vi "Shooter Pneumatics.vi"(10 "Boolean":bool, 11 "Enum":enum16{"Start", "Run", "End"}(ring)=enum."Run") -> (3 "Shooter Angle":T1)   [LabVIEW 2012]
uses:
  <vilib>/Rock Robotics/WPI/Solenoid/WPI_SolenoidChannel.ctl
  <vilib>/Rock Robotics/SystemInterfaces/Typedef/FPGA_TypedefSolenoidModule.ctl
  <vilib>/Rock Robotics/WPI/Solenoid/WPI_SolenoidValue.ctl
  <vilib>/Rock Robotics/WPI/Solenoid/WPI_SolenoidOpenDouble.vi
  <vilib>/Rock Robotics/WPI/Solenoid/WPI_SolenoidSetEnum.vi
panel:
  in  "Solenoid Module 1":T4={"Shoot FWD"=enum."Solenoid 1", "Shoot REV"=enum."Solenoid 2", "Climber"=enum."Solenoid 3", "Climber"=enum."Solenoid 4", "Arm Lock"=enum."Solenoid 5", "Unassigned"=enum."Solenoid 6", "Color"=enum."Solenoid 7", "Unassigned"=enum."Solenoid 8", "Module"=enum."Solenoid Module 1"}
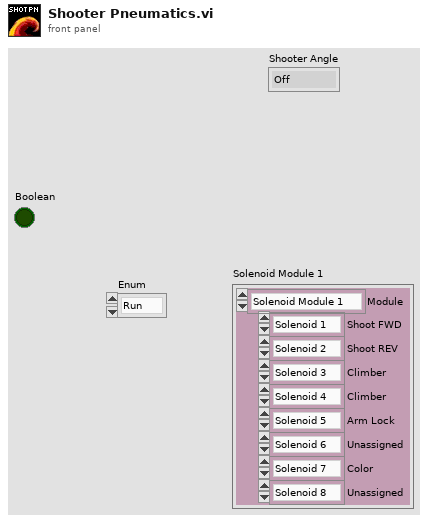
[diagram p1: front panel]
types:
  T1 = typedef "WPI_SolenoidValue.ctl" = enum16{"Off", "On", "Forward", "Reverse"}
  T2 = typedef "WPI_SolenoidChannel.ctl" = enum8{"Solenoid 1", "Solenoid 2", "Solenoid 3", "Solenoid 4", "Solenoid 5", "Solenoid 6", "Solenoid 7", "Solenoid 8", "Invalid"}
  T3 = typedef "FPGA_TypedefSolenoidModule.ctl" = enum16{"Solenoid Module 1", "Solenoid Module 2"}
  T4 = cluster{"Shoot FWD":T2, "Shoot REV":T2, "Climber":T2, "Climber":T2, "Arm Lock":T2, "Unassigned":T2, "Color":T2, "Unassigned":T2, "Module":T3}
  T5 = typedef "WPI_SolenoidDevRef.ctl" = cluster{"DevStatus":errorcluster, "Solenoid Module":T3, "Forward Solenoid Channel":T2, "Reverse Solenoid Channel":T2}
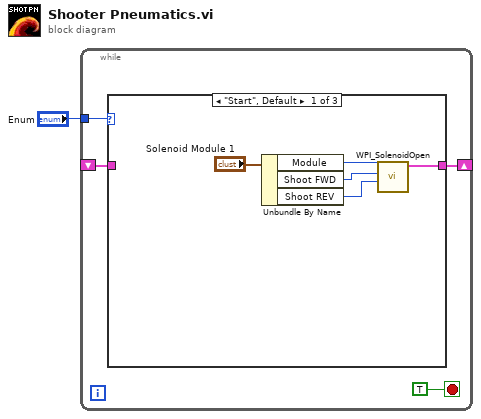
[diagram p0: block diagram]
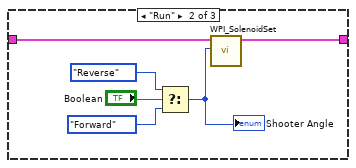
[diagram p2: hidden frame]
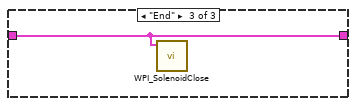
[diagram p3: hidden frame]
diagram:
  n1 = while {
    shift-right: [w5] -> _
    shift-left: _ -> [w3]
    tunnel: "Enum" -> [w4]
    stop <- TRUE stop-if-true
    n2 = case shown="\"Start\", Default" w4 {
      tunnel: [w10 w16 w17] -> w5
      tunnel: w3 -> [_ w15 w17]
      frame "Start", Default {
        n3 = Unbundle By Name("Solenoid Module 1") -> ("Module"=w9:T3, "Shoot FWD"=w8:T2, "Shoot REV"=w7:T2)
        n4 = call-poly <vilib>:"WPI_SolenoidOpen.vi"("Reverse Solenoid Channel"=w7, "Forward Solenoid Channel"=w8, "Solenoid Module (Module 1)"=w9) -> ("SolenoidDevRef"=w10:T5)  [unwired: 7 in, 1 out]
      }
      frame "Run" {
        n5 = Select(t=WPI_SolenoidValue."Reverse" ("Value"), s="Boolean", f=WPI_SolenoidValue."Forward" ("Value")) -> (s? t:f=w11:T1)
        "Shooter Angle" <- w11
        n6 = call-poly <vilib>:"WPI_SolenoidSet.vi"("Value"=w11, "SolenoidDevRef"=w15) -> ("SolenoidDevRef"=w16:T5)  [unwired: 8 in, 1 out]
      }
      frame "End" {
        n7 = call <vilib>:"WPI_SolenoidClose.vi"("SolenoidDevRef"=w17) -> ()  [unwired: 10 in, 1 out]
      }
    }
  }
